vi "SeqWrite.vi"(8 "error in (no error)":errorcluster, 10 "Seqn in":refnum<class "Sequence.lvclass">, 11 "File in":path) -> (0 "error out":errorcluster)   [LabVIEW 2012, in "Sequence.lvclass"]
uses:
  Sequence.lvclass
  Cohort.lvclass
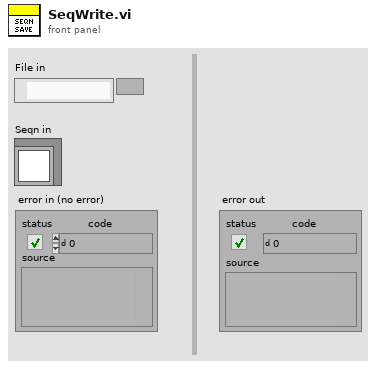
[diagram p1: front panel]
types:
  T1 = enum16{"open", "replace", "create", "open or create", "replace or create", "replace or create with confirmation"}
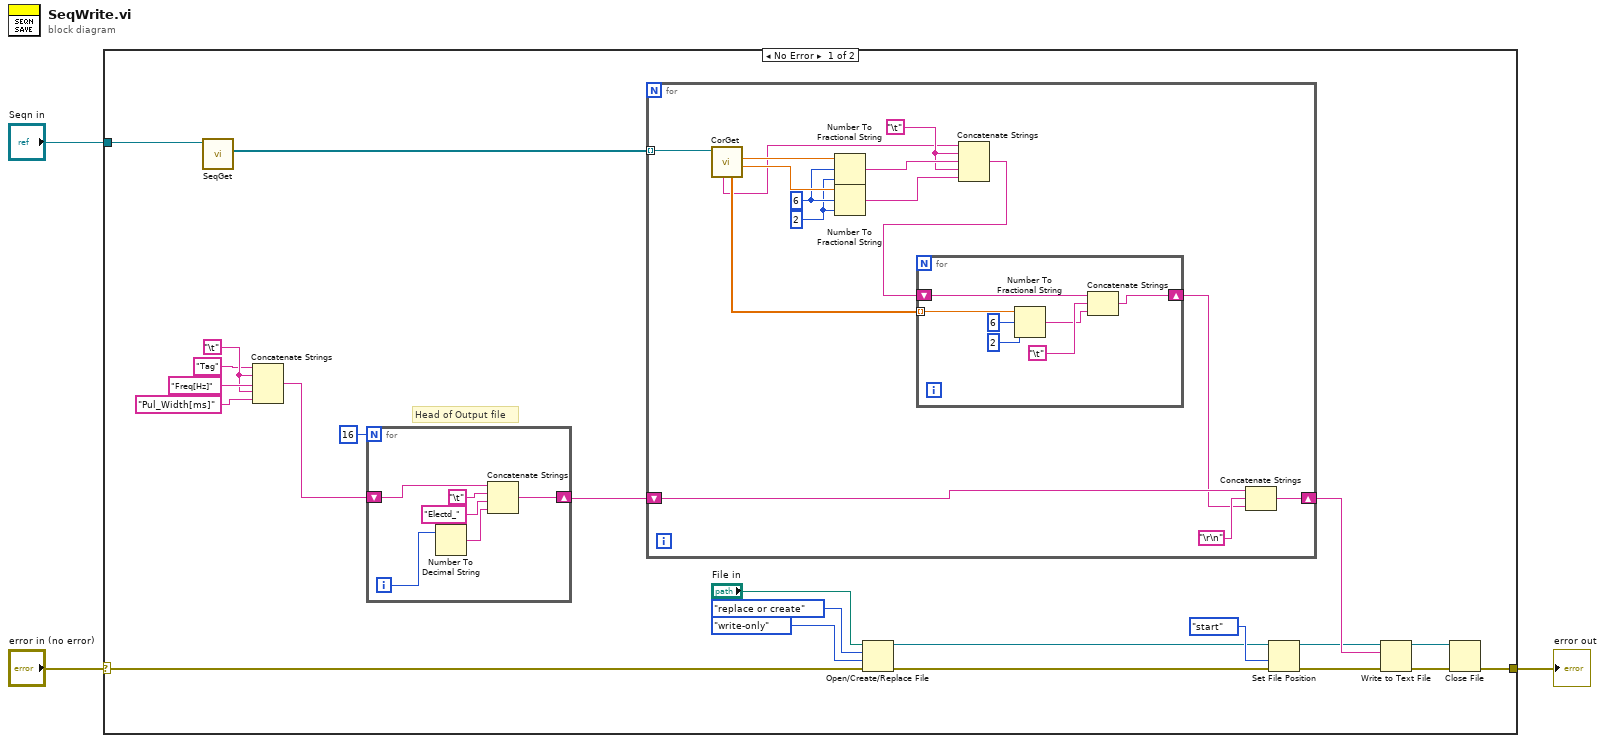
[diagram p0: block diagram]
diagram:
  n1 = case shown="No Error" "error in (no error)" {
    selector: "error in (no error)" -> [w12 w54]
    tunnel: "Seqn in" -> [w25 _]
    tunnel: [w5 w54] -> w2
    frame No Error {
      w14 = "\t"
      # "Head of Output file"
      n2 = call-dynamic "SeqGet.vi"("Sequence in"=w25) -> ("Cohorts"=w24:refnum<class "Cohort.lvclass">[])  [unwired: 7 in, 3 out]
      n3 = Concatenate Strings("Tag", w14, "Freq[Hz]", w14, "Pul_Width[ms]") -> (w19:string)
      n4 = for {
        N: 16 -> [_]
        shift-right: [w28] -> w20
        shift-left: w19 -> [w27]
        i -> [w26]
        n5 = Number To Decimal String(number=w26) -> (decimal integer string=w29:string)  [unwired: 1 in]
        n6 = Concatenate Strings(w27, "\t", "Electd_", w29) -> (w28:string)
      }
      n7 = for {
        tunnel: w24 -> [w46] mode=indexing
        shift-right: [w40] -> w23
        shift-left: w20 -> [w41]
        w33 = "\t"
        w34 = i16 2 ("precision (6)")
        w35 = i16 6 ("width (-)")
        n8 = call-dynamic "CorGet.vi"("Cohort in"=w46) -> ("Pulse Width [ms]"=w45:sgl, "Pulse Frequency [Hz]"=w37:sgl, "Amplitude"=w44:sgl[], "COR Tag"=w32:string)  [unwired: 6 in, 1 out]
        n9 = Number To Fractional String(number=w37, width (-)=w35, precision (6)=w34) -> (F-format string=w36:string)  [unwired: 1 in]
        n10 = Number To Fractional String(number=w45, width (-)=w35, precision (6)=w34) -> (F-format string=w43:string)  [unwired: 1 in]
        n11 = Concatenate Strings(w32, w33, w36, w33, w43) -> (w42:string)
        n12 = for {
          tunnel: w44 -> [w53] mode=indexing
          shift-right: [w50] -> w38
          shift-left: w42 -> [w49]
          n13 = Number To Fractional String(number=w53, width (-)=i16 6, precision (6)=i16 2) -> (F-format string=w47:string)  [unwired: 1 in]
          n14 = Concatenate Strings(w49, "\t", w47) -> (w50:string)
        }
        n15 = Concatenate Strings(w41, "\r\n", w38) -> (w40:string)
      }
      n16 = Open/Create/Replace File(file path (use dialog)="File in", error in=w12, operation (0:open)=T1."replace or create", access (0:read/write)=enum16{"read/write", "read-only", "write-only"}."write-only") -> (refnum out=w10:refnum<file>, error out=w11:errorcluster)  [unwired: 2 in, 1 out]
      n17 = Set File Position(refnum=w10, from (0:start)=enum16{"start", "end", "current"}."start", error in=w11) -> (refnum out=w16:refnum<file>, error out=w17:errorcluster)  [unwired: 1 in]
      n18 = Write to Text File(file (use dialog)=w16, text=w23, error in=w17) -> (refnum out=w4:refnum<file>, error out=w6:errorcluster)  [unwired: 1 in, 1 out]
      n19 = Close File(refnum=w4, error in=w6) -> (error out=w5:errorcluster)  [unwired: 1 out]
    }
    frame Error {
    }
  }
  "error out" <- w2
